vi "B2G2_host_db_logging.vi"() -> ()   [LabVIEW 2011]
uses:
  B2G2_host_db_log_vars.ctl
  <vilib>/addons/database/Connection.llb/Conn ObjectReference.ctl
  Output - Cluster b2g2.ctl
  <vilib>/Platform/TimedLoop/XDataNode/timing_clust.ctl
  <vilib>/Platform/TimedLoop/XDataNode/nitl_modes.ctl
  <vilib>/Platform/TimedLoop/XDataNode/wakeup.ctl
  <vilib>/Platform/TimedLoop/XDataNode/XDataNode.xnode
  <vilib>/Platform/TimedLoop/XDataNode/XDNodeRunTimeDep.lvlib
  <vilib>/addons/database/NI_Database_API.lvlib
  <userlib>/_JGCODE/error_logger/_error_logger.llb/ErrorLogger.lvclass
panel:
  out "target connection":bool
  out "db connection":bool
  in  "prefix for tables":string(combo)="B2G2"
  in  "interval [s]":u32=10 min=1 step=1
  in  "path":path
  in  "stop":bool caption="EXIT"
  # "B2G 2 DB Logging"
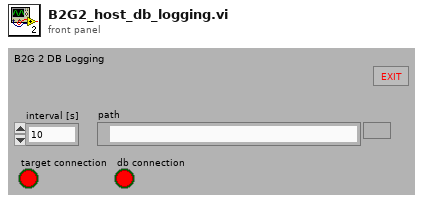
[diagram p1: front panel]
types:
  T1 = typedef "Output - Cluster b2g2.ctl" = cluster{"DFS-1 [dl]":u64, "FS-3 [l]":dbl, "DFS-1 [l/min]":dbl, "DS-1 [bar]":dbl, "V-10 ZU":bool, "V-14 ZU":bool, "FS-1 [l]":dbl, "FS-2 [l]":dbl, "TS-4 [°C]":dbl, "HS-1":bool, "V-13 [%]":u8, "V-15 [%]":u8, "P-4 [%]":u8, "Dosierung":bool, "MR Max Füllstand":bool, "MR Min Füllstand":bool, "Dosiermenge [l]":sgl, "V-14 AUF":bool, "V-10 AUF":bool, "T-1 Max Füllstand":bool, "T-1 Min Füllstand":bool, "T-2 Max Füllstand":bool, "T-2 Min Füllstand":bool, "pHS-1 [pH]":dbl, "P-4 RUN":bool, "V-33 AUF":bool, "V-33 ZU":bool, "V-34 AUF":bool, "V-34 ZU":bool, "P-4 ERR":bool, "TS-5 [°C]":dbl, "V-35 AUF":bool, "V-35 ZU":bool, "P-9 RUN":bool}
  T2 = typedef "B2G2_host_db_log_vars.ctl" = cluster{"db timing":i64, "DFS-1":u64, "db reference":T3, "P4 RUN":bool, "db logging":bool, "data refnum":refnum<k21>, "feeding":bool, "feeding start volume":u64, "feeding start time":timestamp, "flashing":bool, "flashing start volume":u64, "flashing start time":timestamp, "V-33":bool, "V-34":bool, "V-15":u8, "V-13":u8, "P4 ERR":bool, "V-14":bool, "V-10":bool, "prefix":string, "V-35":bool, "output cluster reading time":timestamp, "HS1":bool, "P9 RUN":bool, "db connection":bool}
  T3 = typedef "NI_Database_API.lvlib/Conn ObjectReference.ctl" = refnum<k1>
  T4 = typedef "XDNodeRunTimeDep.lvlib/timing_clust.ctl" = cluster{"Expected End [f-1]":u64, "Actual End [f-1]":u64, "Finished Late? [f-1]":bool, "Expected End [i-1]":u64, "Actual End [i-1]":u64, "Finished Late? [i-1]":bool, "Expected Start [i]":u64, "Actual Start [i]":u64, "Expected Start [f]":u64, "Actual Start [f]":u64, "Source Name":string, "Structure Name":string, "Period":i64, "Deadline":i64, "Offset":i64, "Start":i64, "Priority":i32, "Timeout":i32, "Mode":T5, "Wakeup Reason":T6, "Error":errorcluster, "Source Type":string, "Secondary Source Type":string, "Global End Time":u64, "Global Start Time":u64, "Frame Duration":u64, "Iteration Duration":u64, "Assigned CPU":i32, "I/O Scan Engine Mode":u32}
  T5 = typedef "XDNodeRunTimeDep.lvlib/nitl_modes.ctl" = enum32{"No Change", "Process missed periods, maintain original phase", "Discard missed periods, maintain original phase", "Process missed periods, ignore original phase", "Discard missed periods, ignore original phase"}
  T6 = typedef "XDNodeRunTimeDep.lvlib/wakeup.ctl" = enum32{"Normal", "Aborted", "Asynchronous wakeup", "Timing source error", "Timed loop error", "Timeout"}
  T7 = enum32{"invalid app kind", "Development System", "Run Time System", "Student Edition", "Embedded LabVIEW", "Evaluation", "Custom"}
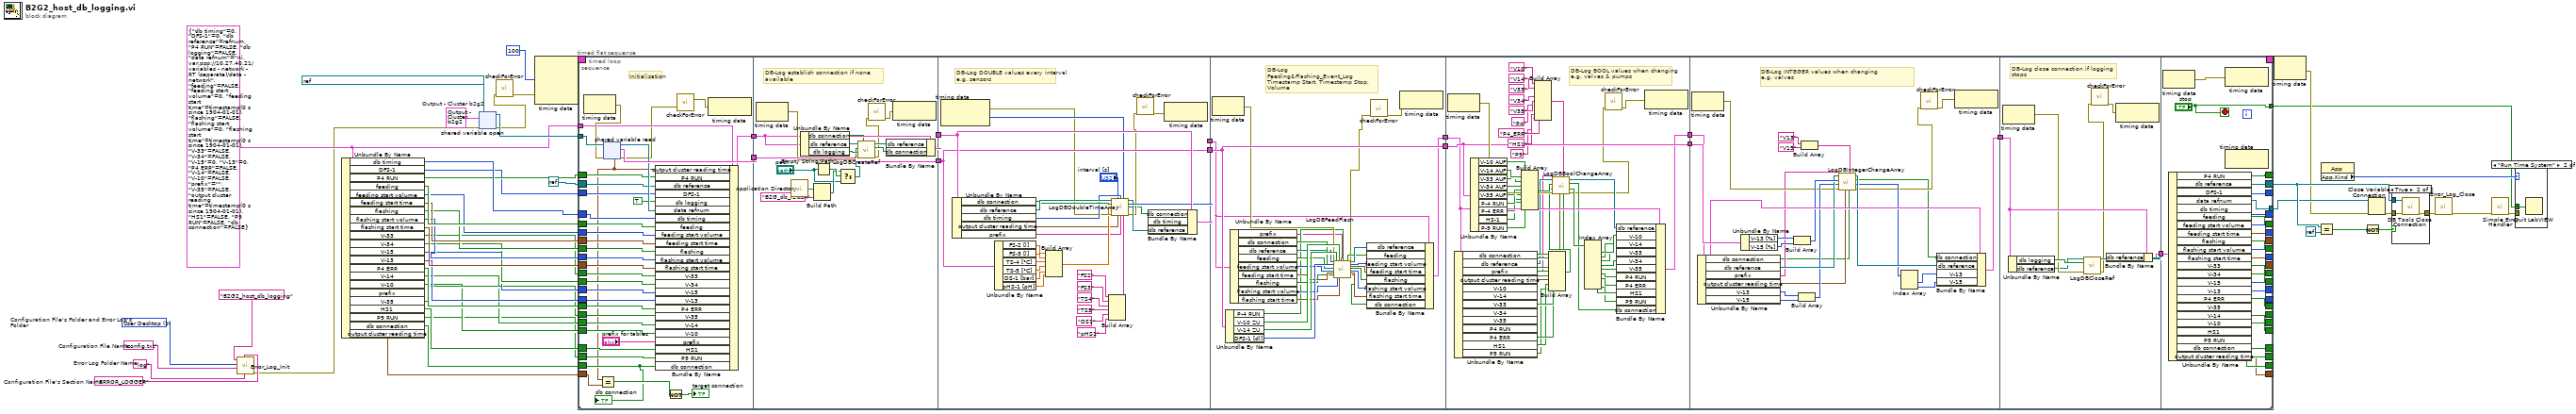
[diagram p0: block diagram]
diagram:
  w29 = "ERROR_LOGGER"  # Configuration File's Section Name
  w30 = "config.txt"  # Configuration File Name
  w31 = "log"  # Error Log Folder Name
  w32 = 1 items=["User Home", "User Desktop", "User Documents", "User Application Data", "User Preferences", "User Temporary", "Public Documents", "Public Application Data", "Public Preferences", "System Core Libraries", "System Installed Libraries", "Application Files", "Boot Volume Root"]  # Configuration File's Folder and Error Log's Folder
  w41 = T1 {"DFS-1 [dl]"=0, "FS-3 [l]"=0.0, "DFS-1 [l/min]"=0.0, "DS-1 [bar]"=0.0, "V-10 ZU"=FALSE, "V-14 ZU"=FALSE, "FS-1 [l]"=0.0, "FS-2 [l]"=0.0, "TS-4 [°C]"=0.0, "HS-1"=FALSE, "V-13 [%]"=0, "V-15 [%]"=0, "P-4 [%]"=0, "Dosierung"=FALSE, "MR Max Füllstand"=FALSE, "MR Min Füllstand"=FALSE, "Dosiermenge [l]"=0.0, "V-14 AUF"=FALSE, "V-10 AUF"=FALSE, "T-1 Max Füllstand"=FALSE, "T-1 Min Füllstand"=FALSE, "T-2 Max Füllstand"=FALSE, "T-2 Min Füllstand"=FALSE, "pHS-1 [pH]"=0.0, "P-4 RUN"=FALSE, "V-33 AUF"=FALSE, "V-33 ZU"=FALSE, "V-34 AUF"=FALSE, "V-34 ZU"=FALSE, "P-4 ERR"=FALSE, "TS-5 [°C]"=0.0, "V-35 AUF"=FALSE, "V-35 ZU"=FALSE, "P-9 RUN"=FALSE}  # Output - Cluster b2g2
  w33 = T2 {"db timing"=0, "DFS-1"=0, "db reference"=refnum, "P4 RUN"=FALSE, "db logging"=FALSE, "data refnum"="ni.var.psp://10.27.40.21/variables - network - RT (separate)/data - network", "feeding"=FALSE, "feeding start volume"=0, "feeding start time"=timestamp(0 s since 1904-01-01), "flashing"=FALSE, "flashing start volume"=0, "flashing start time"=timestamp(0 s since 1904-01-01), "V-33"=FALSE, "V-34"=FALSE, "V-15"=0, "V-13"=0, "P4 ERR"=FALSE, "V-14"=FALSE, "V-10"=FALSE, "prefix"="", "V-35"=FALSE, "output cluster reading time"=timestamp(0 s since 1904-01-01), "HS1"=FALSE, "P9 RUN"=FALSE, "db connection"=FALSE} ("log vars")
  n1 = call "Error_Log_Init.vi"("Error Log Folder Name"=w31, "Configuration File's Section Name"=w29, "Configuration File Name"=w30, "Configuration File's Folder and Error Log's Folder"=w32, "Application Name (Application)"="B2G2_host_db_logging") -> ("error out"=w27:errorcluster)  [unwired: 6 in]
  n2 = Unbundle By Name(w33) -> ("db timing"=w26:i64, "DFS-1"=w24:u64, "P4 RUN"=w25:bool, "feeding"=w23:bool, "feeding start volume"=w21:u64, "feeding start time"=w20:timestamp, "flashing"=w18:bool, "flashing start volume"=w17:u64, "flashing start time"=w19:timestamp, "V-33"=w16:bool, "V-34"=w15:bool, "V-15"=w14:u8, "V-13"=w13:u8, "P4 ERR"=w12:bool, "V-14"=w10:bool, "V-10"=w9:bool, "V-35"=w11:bool, "HS1"=w8:bool, "P9 RUN"=w7:bool, "db connection"=w22:bool, "output cluster reading time"=w6:timestamp)  [unwired: 1 out]
  n3 = shared-variable-open(refnum<k21> "ni.var.psp://10.27.40.25/variables - b2g2/data - network b2g2" ("output variable"), w27, w41) -> (w42:refnum<k21>, w5:errorcluster)  [unwired: 1 in]
  n4 = call <userlib>:"checkForError.vi"("Error In"=w5) -> ("error out"=w4:errorcluster)  [unwired: 9 in, 1 out]
  n5 = node-c288(i64 100 ("Period"), w4) -> (w49:T4)  [unwired: 2 in]
  n6 = timed-loop {
    timing: w49 -> [_]
    timing-out: [_] -> w48
    shift-right: [w97] -> _
    shift-left: w26 -> [w57]
    tunnel: w33 -> [w96]
    shift-right: [w95] -> _
    shift-left: w24 -> [w88]
    shift-right: [w94] -> w43
    shift-left: refnum<k0> refnum -> [w93]
    shift-right: [w92] -> _
    shift-left: w25 -> [w91]
    tunnel: w42 -> [w90]
    tunnel: [w89] -> w39
    shift-right: [w87] -> _
    shift-left: w23 -> [w86]
    shift-right: [w85] -> _
    shift-left: w18 -> [w84]
    shift-right: [w83] -> _
    shift-left: w21 -> [w54]
    shift-right: [w82] -> _
    shift-left: w17 -> [w53]
    shift-right: [w81] -> _
    shift-left: w19 -> [w80]
    shift-right: [w79] -> _
    shift-left: w20 -> [w78]
    shift-right: [w77] -> _
    shift-left: w14 -> [w71]
    shift-right: [w76] -> _
    shift-left: w13 -> [w70]
    shift-right: [w75] -> _
    shift-left: w15 -> [w72]
    shift-right: [w74] -> _
    shift-left: w16 -> [w73]
    shift-right: [w69] -> _
    shift-left: w12 -> [w68]
    shift-right: [w67] -> _
    shift-left: w10 -> [w64]
    shift-right: [w66] -> _
    shift-left: w9 -> [w65]
    shift-right: [w63] -> _
    shift-left: w11 -> [w52]
    tunnel: [w62] -> w34
    shift-right: [w61] -> _
    shift-left: w8 -> [w60]
    shift-right: [w59] -> _
    shift-left: w7 -> [w58]
    shift-right: [w56] -> _
    shift-left: w22 -> [w55]
    shift-right: [w51] -> _
    shift-left: w6 -> [w50]
    stop <- "stop" stop-if-true
    n7 = timed-sequence {
      timing: _ -> [_]
      timing-out: _ -> [_]
      tunnel: [w157] -> w97
      tunnel: w96 -> [w156]
      tunnel: [w155] -> w95
      tunnel: [w154] -> w94
      tunnel: w93 -> [w153]
      tunnel: [w152] -> w92
      tunnel: w91 -> [w151]
      tunnel: w90 -> [w146]
      tunnel: [w145] -> w89
      tunnel: w88 -> [w144]
      tunnel: [w141] -> w87
      tunnel: w86 -> [w140]
      tunnel: [w139] -> w85
      tunnel: w84 -> [w138]
      tunnel: [w137] -> w83
      tunnel: [w136] -> w82
      tunnel: [w135] -> w81
      tunnel: w80 -> [w134]
      tunnel: [w133] -> w79
      tunnel: w78 -> [w132]
      tunnel: [w129] -> w77
      tunnel: [w128] -> w76
      tunnel: [w127] -> w75
      tunnel: [w126] -> w74
      tunnel: w73 -> [w125]
      tunnel: w72 -> [w124]
      tunnel: w71 -> [w123]
      tunnel: w70 -> [w122]
      tunnel: [w118] -> w69
      tunnel: w68 -> [w117]
      tunnel: [w116] -> w67
      tunnel: [w115] -> w66
      tunnel: w65 -> [w114]
      tunnel: w64 -> [w113]
      tunnel: [w112] -> w63
      tunnel: [w110] -> w62
      tunnel: [w109] -> w61
      tunnel: w60 -> [w108]
      tunnel: [w107] -> w59
      tunnel: w58 -> [w106]
      tunnel: w57 -> [w105]
      tunnel: [w104] -> w56
      tunnel: w55 -> [w103]
      tunnel: w54 -> [w102]
      tunnel: w53 -> [w101]
      tunnel: w52 -> [w100]
      tunnel: [w99] -> w51
      tunnel: w50 -> [w98]
      n8 = timed-flat-sequence {
        tunnel: [w190] -> w150
        tunnel: w156 -> [w177]
        tunnel: [w176] -> w148
        tunnel: w153 -> [w168]
        tunnel: w151 -> [w178]
        tunnel: w146 -> [w192]
        tunnel: w144 -> [w169]
        tunnel: w140 -> [w180]
        tunnel: w138 -> [w183]
        tunnel: w134 -> [w185]
        tunnel: w132 -> [w182]
        tunnel: w125 -> [w186]
        tunnel: w124 -> [w187]
        tunnel: w123 -> [w188]
        tunnel: w122 -> [w189]
        tunnel: w117 -> [w175]
        tunnel: w114 -> [w173]
        tunnel: w113 -> [w174]
        tunnel: w108 -> [w167]
        tunnel: w106 -> [w166]
        tunnel: w105 -> [w170]
        tunnel: w103 -> [w162]
        tunnel: w102 -> [w181]
        tunnel: w101 -> [w184]
        tunnel: w100 -> [w171]
        tunnel: w98 -> [w160]
        tunnel: w150 -> [w214]
        tunnel: [w214] -> w149
        tunnel: w148 -> [w211]
        tunnel: [w210] -> w147
        tunnel: w149 -> [w235]
        tunnel: [w235] -> w143
        tunnel: w147 -> [w248]
        tunnel: [w249] -> w142
        tunnel: w143 -> [w282]
        tunnel: [w282] -> w131
        tunnel: w142 -> [w271]
        tunnel: [w277] -> w130
        tunnel: w131 -> [w338]
        tunnel: [w338] -> w121
        tunnel: w130 -> [w323]
        tunnel: [w324] -> w120
        tunnel: w121 -> [w367]
        tunnel: w120 -> [w364]
        tunnel: [w368] -> w119
        tunnel: w119 -> [w380]
        tunnel: [w376] -> w111
        tunnel: [w394] -> w157
        tunnel: [w393] -> w155
        tunnel: [w392] -> w154
        tunnel: [w411] -> w152
        tunnel: [w410] -> w145
        tunnel: [w409] -> w141
        tunnel: [w406] -> w139
        tunnel: [w408] -> w137
        tunnel: [w405] -> w136
        tunnel: [w404] -> w135
        tunnel: [w407] -> w133
        tunnel: [w401] -> w129
        tunnel: [w400] -> w128
        tunnel: [w402] -> w127
        tunnel: [w403] -> w126
        tunnel: [w399] -> w118
        tunnel: [w398] -> w116
        tunnel: [w397] -> w115
        tunnel: [w396] -> w112
        tunnel: w111 -> [w395]
        tunnel: ["stop"] -> w110
        tunnel: [w390] -> w109
        tunnel: [w389] -> w107
        tunnel: [w388] -> w104
        tunnel: [w387] -> w99
        frame #0 {
          # "Initialisation"
          n9 = node-c288() -> (w191:errorcluster)  [unwired: 1 in]
          n10 = shared-variable-read(w192, w191) -> (w179:refnum<k21>, w159:errorcluster, w190:T1, w161:timestamp)
          n11 = Equal?(x=w161, y=w160) -> (x = y?=w163:bool)
          n12 = Bundle By Name(cluster=w177, "output cluster reading time"=w161, "P4 RUN"=w178, "db reference"=w168, "DFS-1"=w169, "db logging"=TRUE ("db"), "data refnum"=w179, "db timing"=w170, "feeding"=w180, "feeding start volume"=w181, "feeding start time"=w182, "flashing"=w183, "flashing start volume"=w184, "flashing start time"=w185, "V-33"=w186, "V-34"=w187, "V-15"=w188, "V-13"=w189, "P4 ERR"=w175, "V-35"=w171, "V-14"=w174, "V-10"=w173, "prefix"="prefix for tables", "HS1"=w167, "P9 RUN"=w166, "db connection"=w162) -> (w176:T2)
          n13 = Not(x=w163) -> (.not. x?=→"target connection":bool)
          n14 = call <userlib>:"checkForError.vi"("Error In"=w159) -> ("error out"=w158:errorcluster)  [unwired: 9 in, 1 out]
          n15 = node-c288(w158) -> ()  [unwired: 1 out]
          "db connection" <- w162
        }
        frame #1 {
          # "DB-Log establish connection if none available"
          n16 = node-c288() -> (w212:errorcluster)  [unwired: 1 in]
          n17 = call <vilib>:"Application Directory.vi"() -> ("Application Directory"=w205:path)
          n18 = Unbundle By Name(w211) -> ("db connection"=w201:bool, "db reference"=w213:T3, "db logging"=w208:bool)
          n19 = Build Path(base path=w205, name or relative path="B2G_db_rz.dsn" ("Name of ini file 2")) -> (appended path=w206:path)
          n20 = Empty String/Path?(string/path="path") -> (empty?=w207:bool)
          n21 = Select(t=w206, s=w207, f="path") -> (s? t:f=w202:path)
          n22 = call "LogDBCreateRef.vi"("db connection"=w201, "error in (no error)"=w212, "db"=w208, "Pfad in"=w202, "Refnum in"=w213) -> ("error out"=w199:errorcluster, "db connection"=w200:bool, "Refnum out"=w209:T3)  [unwired: 4 in]
          n23 = call <userlib>:"checkForError.vi"("Error In"=w199) -> ("error out"=w198:errorcluster)  [unwired: 9 in, 1 out]
          n24 = Bundle By Name(cluster=w211, "db reference"=w209, "db connection"=w200) -> (w210:T2)
          n25 = node-c288(w198) -> ()  [unwired: 1 out]
        }
        frame #2 {
          # "DB-Log DOUBLE values every interval\ne.g. sensors"
          n26 = node-c288() -> (w227:errorcluster, w230:i64)  [unwired: 1 in]
          n27 = Unbundle By Name(w248) -> ("db connection"=w233:bool, "db reference"=w234:T3, "db timing"=w232:i64, "output cluster reading time"=w223:timestamp, "prefix"=w224:string)
          n28 = Unbundle By Name(w235) -> ("FS-2 [l]"=w236:dbl, "FS-3 [l]"=w237:dbl, "TS-4 [°C]"=w238:dbl, "TS-5 [°C]"=w239:dbl, "DS-1 [bar]"=w240:dbl, "pHS-1 [pH]"=w241:dbl)
          n29 = Build Array(w236, w237, w238, w239, w240, w241) -> (w226:dbl[])
          n30 = Build Array("FS2" ("table"), "FS3" ("table"), "TS4" ("table"), "TS5" ("table"), "DS1" ("table"), "pHS1" ("table")) -> (w225:string[])
          n31 = call "LogDBDoubleTimeArray.vi"("Refnum in"=w234, "db Interval [s]"="interval [s]", "db timing"=w232, "Actual Start [f] in"=w230, "db connection"=w233, "values"=w226, "error in (no error)"=w227, "Time Stamp"=w223, "prefix"=w224, "names"=w225) -> ("Refnum out"=w228:T3, "Actual Start [f] out"=w229:i64, "db connection"=w220:bool, "error out"=w222:errorcluster)  [unwired: 2 in]
          n32 = call <userlib>:"checkForError.vi"("Error In"=w222) -> ("error out"=w221:errorcluster)  [unwired: 9 in, 1 out]
          n33 = Bundle By Name(cluster=w248, "db connection"=w220, "db timing"=w229, "db reference"=w228) -> (w249:T2)
          n34 = node-c288(w221) -> ()  [unwired: 1 out]
        }
        frame #3 {
          # "DB-Log\nFeeding&Flashing_Event_Log\nTimestamp Start, Timestamp Stop, Volume"
          n35 = node-c288() -> (w278:errorcluster)  [unwired: 1 in]
          n36 = Unbundle By Name(w282) -> ("P-4 RUN"=w260:bool, "V-10 ZU"=w280:bool, "V-14 ZU"=w279:bool, "DFS-1 [dl]"=w281:u64)
          n37 = Unbundle By Name(w271) -> ("prefix"=w259:string, "db connection"=w274:bool, "db reference"=w273:T3, "feeding"=w261:bool, "feeding start volume"=w272:u64, "feeding start time"=w270:timestamp, "flashing"=w262:bool, "flashing start volume"=w264:u64, "flashing start time"=w263:timestamp)
          n38 = call "LogDBFeedFlash.vi"("Refnum in"=w273, "value volume [dl]"=w281, "db connection"=w274, "feeding"=w261, "feeding start volume"=w272, "feeding start time"=w270, "flashing"=w262, "error in"=w278, "valve t-2 close"=w279, "flashing start volume"=w264, "valve t-1 close"=w280, "flashing start time"=w263, "prefix"=w259, "Pump"=w260) -> ("feeding"=w275:bool, "Refnum out"=w276:T3, "feeding start volume"=w268:u64, "feeding start time"=w269:timestamp, "flashing"=w266:bool, "flashing start volume"=w265:u64, "flashing start time"=w267:timestamp, "db connection"=w256:bool, "error out"=w258:errorcluster)  [unwired: 5 in]
          n39 = Bundle By Name(cluster=w271, "db reference"=w276, "feeding"=w275, "feeding start volume"=w268, "feeding start time"=w269, "flashing"=w266, "flashing start volume"=w265, "flashing start time"=w267, "db connection"=w256) -> (w277:T2)
          n40 = call <userlib>:"checkForError.vi"("Error In"=w258) -> ("error out"=w257:errorcluster)  [unwired: 9 in, 1 out]
          n41 = node-c288(w257) -> ()  [unwired: 1 out]
        }
        frame #4 {
          # "DB-Log BOOL values when changing\ne.g. valves & pumps"
          n42 = node-c288() -> (w339:errorcluster)  [unwired: 1 in]
          n43 = Unbundle By Name(w323) -> ("db connection"=w301:bool, "db reference"=w312:T3, "prefix"=w311:string, "output cluster reading time"=w310:timestamp, "V-10"=w322:bool, "V-14"=w321:bool, "V-33"=w320:bool, "V-34"=w319:bool, "V-35"=w318:bool, "P4 RUN"=w317:bool, "P4 ERR"=w316:bool, "HS1"=w299:bool, "P9 RUN"=w291:bool)
          n44 = Unbundle By Name(w338) -> ("V-10 AUF"=w337:bool, "V-14 AUF"=w336:bool, "V-33 AUF"=w335:bool, "V-34 AUF"=w334:bool, "V-35 AUF"=w333:bool, "P-4 RUN"=w298:bool, "P-4 ERR"=w297:bool, "HS-1"=w296:bool, "P-9 RUN"=w294:bool)
          n45 = Build Array(w337, w336, w335, w334, w333, w298, w297, w296, w294) -> (w326:bool[])
          n46 = Build Array("V10" ("table"), "V14" ("table"), "V33" ("table"), "V34" ("table"), "V35" ("table"), "P4" ("table"), "P4_ERR" ("table"), "HS1" ("table"), "P9" ("table")) -> (w327:string[])
          n47 = Build Array(w322, w321, w320, w319, w318, w317, w316, w299, w291) -> (w313:bool[])
          n48 = call "LogDBBoolChangeArray.vi"("db connection"=w301, "names"=w327, "cluster reading time"=w310, "prefix"=w311, "error in (no error)"=w339, "shift reg in"=w313, "values"=w326, "db reference"=w312) -> ("error out"=w289:errorcluster, "shift reg out"=w325:bool[], "db connection"=w290:bool, "db reference out"=w302:T3)
          n49 = Index Array(array=w325) -> (element #1=w309:bool, element #2=w308:bool, element #3=w307:bool, element #4=w306:bool, element #5=w305:bool, element #6=w304:bool, element #7=w303:bool, element #8=w300:bool, element #9=w292:bool)  [unwired: 9 in]
          n50 = call <userlib>:"checkForError.vi"("Error In"=w289) -> ("error out"=w288:errorcluster)  [unwired: 9 in, 1 out]
          n51 = Bundle By Name(cluster=w323, "db reference"=w302, "V-10"=w309, "V-14"=w308, "V-33"=w307, "V-34"=w306, "V-35"=w305, "P4 RUN"=w304, "P4 ERR"=w303, "HS1"=w300, "P9 RUN"=w292, "db connection"=w290) -> (w324:T2)
          n52 = node-c288(w288) -> ()  [unwired: 1 out]
        }
        frame #5 {
          # "DB-Log INTEGER values when changing\ne.g. valves"
          n53 = node-c288() -> (w355:errorcluster)  [unwired: 1 in]
          n54 = Unbundle By Name(w364) -> ("db connection"=w348:bool, "db reference"=w359:T3, "prefix"=w349:string, "output cluster reading time"=w350:timestamp, "V-13"=w358:u8, "V-15"=w357:u8)
          n55 = Unbundle By Name(w367) -> ("V-13 [%]"=w362:u8, "V-15 [%]"=w361:u8)
          n56 = Build Array(w362, w361) -> (w360:u8[])
          n57 = Build Array(w358, w357) -> (w356:u8[])
          n58 = Build Array("V13" ("table"), "V15" ("table")) -> (w363:string[])
          n59 = call "LogDBIntegerChangeArray.vi"("db connection"=w348, "names"=w363, "current time"=w350, "prefix"=w349, "error in (no error)"=w355, "shift reg in"=w356, "values"=w360, "Refnum in"=w359) -> ("error out"=w347:errorcluster, "shift reg out"=w351:u32[], "db connection"=w345:bool, "Refnum out"=w354:T3)
          n60 = Index Array(array=w351) -> (element #1=w353:u32, element #2=w352:u32)  [unwired: 2 in]
          n61 = call <userlib>:"checkForError.vi"("Error In"=w347) -> ("error out"=w346:errorcluster)  [unwired: 9 in, 1 out]
          n62 = Bundle By Name(cluster=w364, "db connection"=w345, "db reference"=w354, "V-13"=w353, "V-15"=w352) -> (w368:T2)
          n63 = node-c288(w346) -> ()  [unwired: 1 out]
        }
        frame #6 {
          # "DB-Log close connection if logging stops"
          n64 = node-c288() -> (w378:errorcluster)  [unwired: 1 in]
          n65 = Unbundle By Name(w380) -> ("db logging"=w379:bool, "db reference"=w377:T3)
          n66 = call "LogDBCloseRef.vi"("error in (no error)"=w378, "enable"=w379, "Refnum in"=w377) -> ("error out"=w375:errorcluster, "Refnum out"=w381:T3)  [unwired: 7 in]
          n67 = call <userlib>:"checkForError.vi"("Error In"=w375) -> ("error out"=w374:errorcluster)  [unwired: 9 in, 1 out]
          n68 = Bundle By Name(cluster=w380, "db reference"=w381) -> (w376:T2)
          n69 = node-c288(w374) -> ()  [unwired: 1 out]
        }
        frame #7 {
          n70 = node-c288() -> (w412:errorcluster)  [unwired: 1 in]
          n71 = Unbundle By Name(w395) -> ("P4 RUN"=w411:bool, "db reference"=w392:T3, "DFS-1"=w393:u64, "data refnum"=w410:refnum<k21>, "db timing"=w394:i64, "feeding"=w409:bool, "feeding start volume"=w408:u64, "feeding start time"=w407:timestamp, "flashing"=w406:bool, "flashing start volume"=w405:u64, "flashing start time"=w404:timestamp, "V-33"=w403:bool, "V-34"=w402:bool, "V-15"=w401:u8, "V-13"=w400:u8, "P4 ERR"=w399:bool, "V-35"=w396:bool, "V-14"=w398:bool, "V-10"=w397:bool, "HS1"=w390:bool, "P9 RUN"=w389:bool, "db connection"=w388:bool, "output cluster reading time"=w387:timestamp)
          n72 = node-c288(w412) -> ()  [unwired: 1 out]
        }
      }
    }
    n73 = node-c288() -> ()  [unwired: 1 in, 1 out]
    n74 = node-c288() -> ()  [unwired: 1 in, 1 out]
  }
  n75 = node-c288(w48) -> (w38:errorcluster)
  n76 = Equal?(x=w43, y=refnum<k0> refnum) -> (x = y?=w46:bool)
  n77 = property class="App"() -> ("App.Kind"=w35:T7)  [unwired: 2 in, 2 out]
  n78 = Not(x=w46) -> (.not. x?=w44:bool)
  n79 = Close Variable Connection(8:w38, 11:w39) -> (0:w37:errorcluster)
  n80 = case shown="True" w44 {
    tunnel: w37 -> [w420 w423]
    tunnel: w43 -> [_ w422]
    tunnel: [w420 w421] -> w3
    frame False {
    }
    frame True {
      n81 = call <vilib>:"DB Tools Close Connection.vi"("error in (no error)"=w423, "connection reference"=w422) -> ("error out"=w421:errorcluster)  [unwired: 5 in]
    }
  }
  n82 = call "Error_Log_Close.vi"("error in (no error)"=w3) -> ("error out"=w2:errorcluster)  [unwired: 10 in]
  n83 = call <vilib>:"Simple Error Handler.vi"("error in (no error)"=w2) -> ("error out"=w1:errorcluster)  [unwired: 4 in, 4 out]
  n84 = case shown="\"Run Time System\"" w35 {
    tunnel: w34 -> [_ w424 _]
    tunnel: w1 -> [_ _ _]
    frame "invalid app kind", Default {
    }
    frame "Run Time System" {
      n85 = Quit LabVIEW(quit? (T)=w424) -> ()
    }
    frame "Development System" {
    }
  }
